vi "Copy Buffer to Image (Default Stride Greyscale).vi"(7 "Image Size":T2, 8 "error in (no error)":errorcluster, 10 "Greyscale Image Destination in":T1, 11 "Buffer":u8[](array[numeric])) -> (0 "error out":errorcluster, 3 "Greyscale Image Destination":T1)   [LabVIEW 2020, in "image.lvlib"]
doc: "Copy the Buffer into the Image Destination.\n\nThe Destination will be resized to acommodate the Buffer's data."
uses:
  image.lvlib
  common/Image Size (Integer).ctl
  Greyscale Image.ctl
  Buffer Information.ctl
  Raw Memory Information Dimension.ctl
  f11fe23a-4bac-4ce6-b593-80dfc143e0fd.vi
  <vilib>/Utility/error.llb/Error Cluster From Error Code.vi
  common/common.lvlib
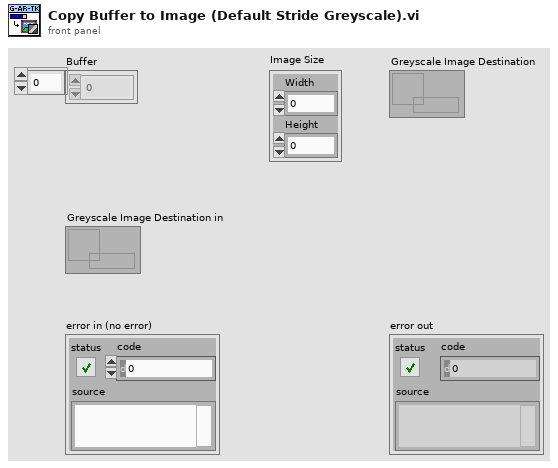
[diagram p1: front panel]
types:
  T1 = typedef "image.lvlib/Greyscale Image.ctl" = refnum<data-value>
  T2 = typedef "common.lvlib/Image Size (Integer).ctl" = cluster{"Width":u16, "Height":u16}
  T3 = typedef "image.lvlib/Buffer Information.ctl" = cluster{"Dimension 0":T4, "Dimension 1":T4}
  T4 = typedef "image.lvlib/Raw Memory Information Dimension.ctl" = cluster{"Size":u16, "Stride":i32}
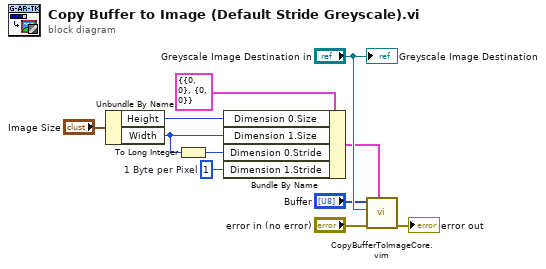
[diagram p0: block diagram]
diagram:
  w4 = 1  # 1 Byte per Pixel
  n1 = Unbundle By Name("Image Size") -> ("Height"=w6:u16, "Width"=w5:u16)
  n2 = To Long Integer(number=w5) -> (32bit integer=w1:i32)
  n3 = Bundle By Name(cluster=T3 {"Dimension 0"={"Size"=0, "Stride"=0}, "Dimension 1"={"Size"=0, "Stride"=0}} ("Buffer Information"), "Dimension 0.Size"=w6, "Dimension 1.Size"=w5, "Dimension 0.Stride"=w1, "Dimension 1.Stride"=w4) -> (w3:T3)
  n4 = call "CopyBufferToImageCore.vim"("Buffer Information"=w3, "error in (no error)"="error in (no error)", "Dst"="Greyscale Image Destination in", "Buffer"="Buffer") -> ("error out"=→"error out":errorcluster)  [unwired: 7 in]
  "Greyscale Image Destination" <- "Greyscale Image Destination in"
